vi "read-first-image.vi"() -> ()   [LabVIEW 2011, in "librir.lvlib"]
uses:
  librir.lvlib
panel:
  in  "pos":i32
  out "pixels":u16[][](array[numeric])
  in  "filename":path
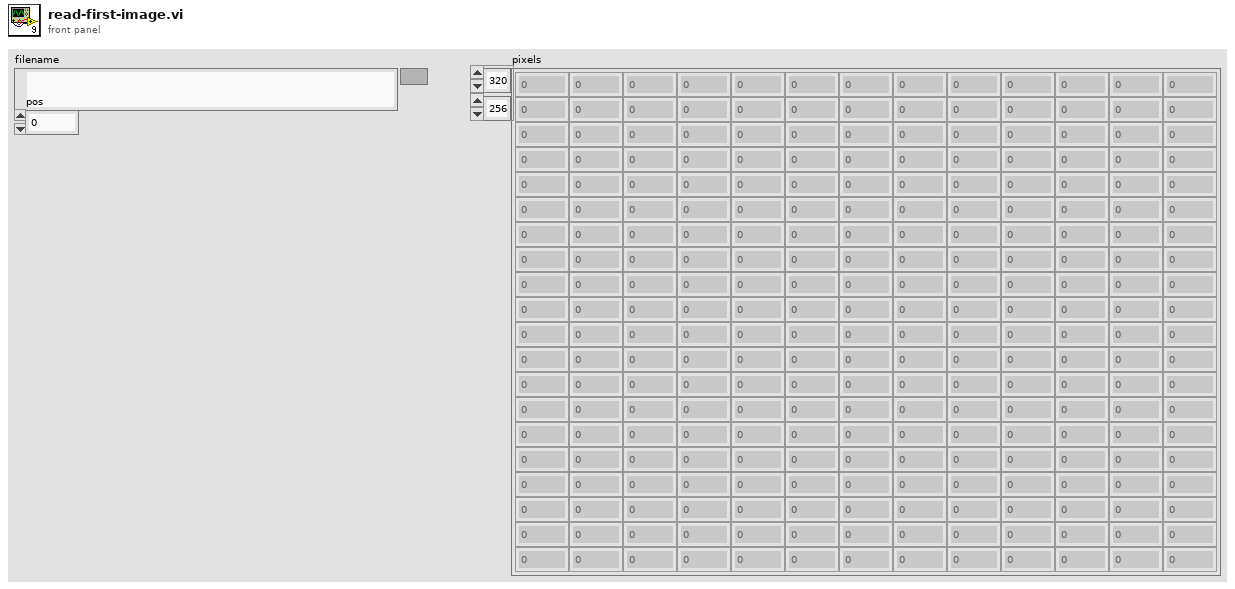
[diagram p1: front panel]
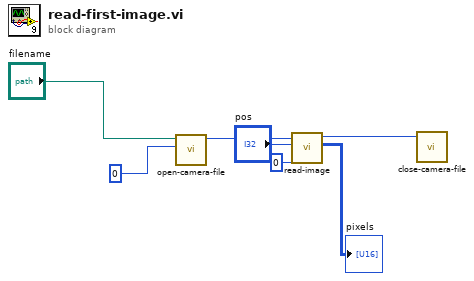
[diagram p0: block diagram]
diagram:
  n1 = call "open-camera-file.vi"("file_format"=0, "filename"="filename") -> ("ir_file_handler"=w5:u64)  [unwired: 9 in]
  n2 = call "read-image.vi"("calibration"=0, "pos"="pos", "ir_file_handler"=w5) -> ("pixels"=→"pixels":u16[][], "ir_file_handler"=w4:u64)  [unwired: 7 in]
  n3 = call "close-camera-file.vi"("ir_file_handler"=w4) -> ()  [unwired: 10 in, 1 out]
